vi "GetGearMainpulatorUpDown.vi"(8 "error in (no error)":errorcluster) -> (0 "error out":errorcluster, 3 "Gear Mainpulator Up Down":enum16{"Up", "Down"}(ring))   [LabVIEW 2016, in "Gear Manipulator.lvclass"]
uses:
  Gear Manipulator.lvclass
  Gear Manipulator.lvclass/Gear Manipulator.ctl
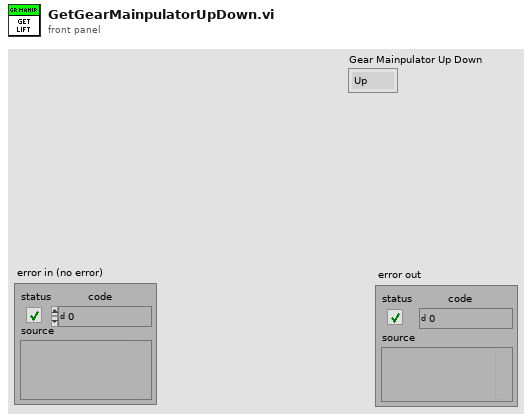
[diagram p1: front panel]
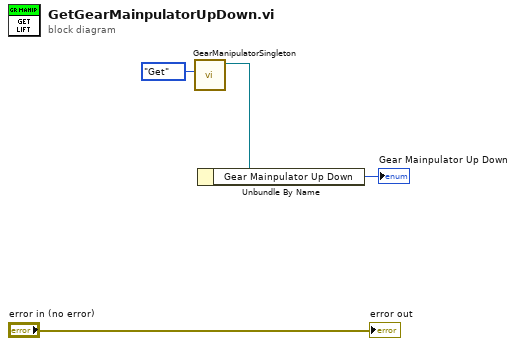
[diagram p0: block diagram]
diagram:
  n1 = call "GearManipulatorSingleton.vi"("Get/Set"=enum16{"Get", "Set"}."Get") -> ("Gear Manipulator.lvclass"=w3:refnum<class "Gear Manipulator.lvclass">)  [unwired: 9 in, 1 out]
  n2 = Unbundle By Name(w3) -> ("Gear Mainpulator Up Down"=→"Gear Mainpulator Up Down":enum16{"Up", "Down"})
  "error out" <- "error in (no error)"
